vi "ring_digital_visible.vi"(8 "error in (no error)":errorcluster, 11 "VI Ref In":refnum<vi>) -> (0 "error out":errorcluster, 3 "VI Ref Out":refnum<vi>)   [LabVIEW 2018]
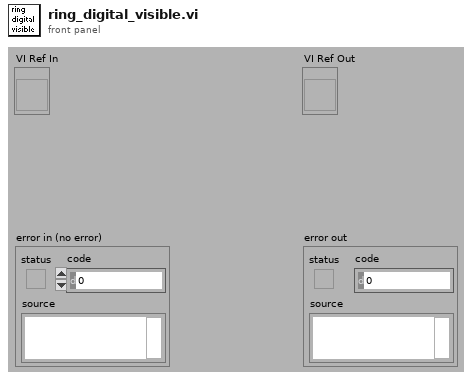
[diagram p1: front panel]
types:
  T1 = typedef "LVRectTypeDef.ctl" = cluster{"Left":i16, "Top":i16, "Right":i16, "Bottom":i16}
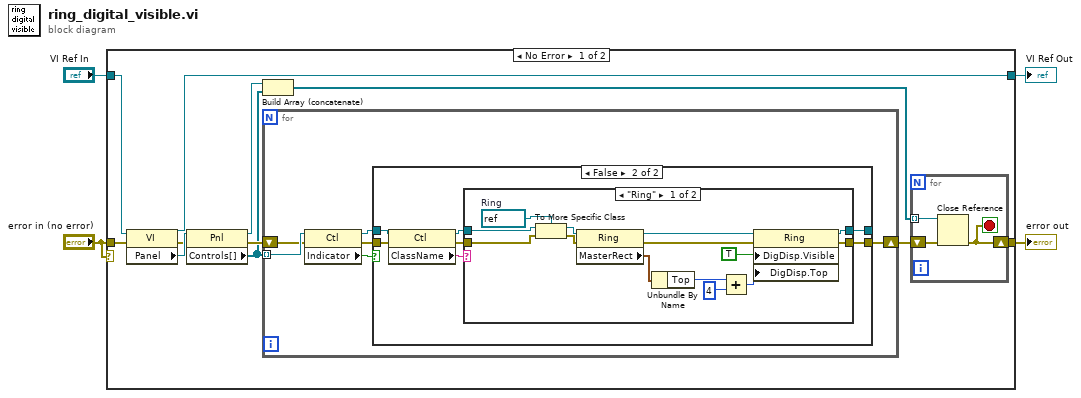
[diagram p0: block diagram]
diagram:
  n1 = case shown="No Error" "error in (no error)" {
    tunnel: [w8 w51] -> w4
    tunnel: "VI Ref In" -> [w7 w51]
    tunnel: "error in (no error)" -> [w6 w50]
    tunnel: [w5 w50] -> w3
    frame No Error {
      n2 = property class="VI"(reference=w7, error in=w6) -> (reference out=w8:refnum<vi>, error out=w14:errorcluster, "Panel"=w15:refnum<vi>)
      n3 = property class="Pnl"(reference=w15, error in=w14) -> (reference out=w12:refnum<vi>, error out=w13:errorcluster, "Controls[]"=w11:refnum<vi>[])
      n4 = Build Array (concatenate)(w12, w11) -> (w10:refnum<vi>[])
      n5 = for {
        tunnel: w11 -> [w24] mode=indexing
        shift-right: [w19] -> w9
        shift-left: w13 -> [w21]
        n6 = property class="Ctl"(reference=w24, error in=w21) -> (reference out=w22:refnum<vi>, error out=w20:errorcluster, "Indicator"=w23:bool)
        n7 = case shown="False" w23 {
          tunnel: w20 -> [w25 w32]
          tunnel: [w25 w30] -> w19
          tunnel: [w26 w29] -> _
          tunnel: w22 -> [w26 w28]
          frame True {
          }
          frame False {
            n8 = property class="Ctl"(reference=w28, error in=w32) -> (reference out=w31:refnum<vi>, error out=w33:errorcluster, "ClassName"=w27:string)
            n9 = case shown="\"Ring\"" w27 {
              tunnel: w31 -> [w46 w48]
              tunnel: w33 -> [w35 w49]
              tunnel: [w44 w49] -> w30
              tunnel: [w45 w48] -> w29
              frame "Ring" {
                w47 = refnum<vi> refnum  # Ring
                n10 = To More Specific Class(target class=w47, reference=w46, error in=w35) -> (specific class reference=w42:refnum<vi>, error out=w34:errorcluster)
                n11 = property class="Ring"(reference=w42, error in=w34) -> (reference out=w41:refnum<vi>, error out=w40:errorcluster, "MasterRect"=w39:T1)
                n12 = Unbundle By Name(w39) -> ("Top"=w37:i16)
                n13 = Add(x=w37, y=i16 4) -> (x+y=w38:i16)
                n14 = property class="Ring"(reference=w41, error in=w40, "DigDisp.Visible"=TRUE ("Digital Display.Visible"), "DigDisp.Top"=w38) -> (reference out=w45:refnum<vi>, error out=w44:errorcluster)
              }
              frame Default {
              }
            }
          }
        }
      }
      n15 = for {
        tunnel: w10 -> [w18] mode=indexing
        shift-right: [w16] -> w5
        shift-left: w9 -> [w17]
        stop <- w16 stop-if-true
        n16 = Close Reference(reference=w18, error in (no error)=w17) -> (error out=w16:errorcluster)
      }
    }
    frame Error {
    }
  }
  "VI Ref Out" <- w4
  "error out" <- w3
